vi "MA-K3BarcodeReader_Initialize.vi"(7 "Timeout(1000ms)":u32=1000, 8 "Error In":errorcluster, 11 "±½½X¾÷¦ê¤f":refnum<visa-resource-name>) -> (0 "Error Out":errorcluster, 3 "VISA Resource":refnum<visa-resource-name>)   [LabVIEW 2019]
uses:
  <vilib>/Instr/_visa.llb/VISA Configure Serial Port (Instr).vi
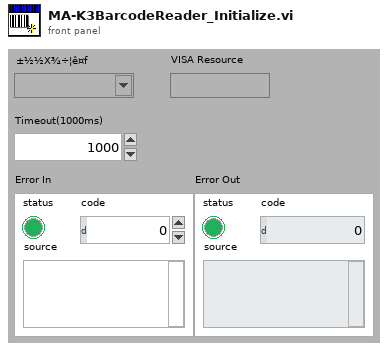
[diagram p1: front panel]
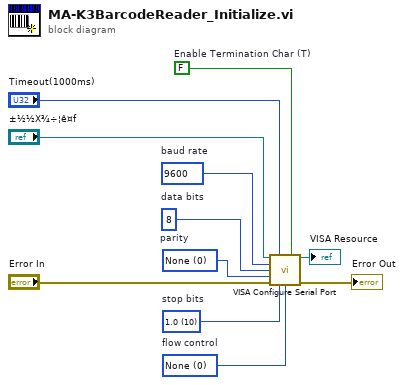
[diagram p0: block diagram]
diagram:
  w10 = u16 0 items=["None"=0, "XON/XOFF"=1, "RTS/CTS"=2, "DTR/DSR"=4]  # flow control
  w9 = u16 10 items=["1.0"=10, "1.5"=15, "2.0"=20]  # stop bits
  w7 = u16 0 items=["None", "Odd", "Even", "Mark", "Space"]  # parity
  w11 = u16 8  # data bits
  w6 = u32 9600  # baud rate
  w8 = FALSE  # Enable Termination Char (T)
  n1 = call-poly "VISA Configure Serial Port"("VISA resource name"="±½½X¾÷¦ê¤f", "timeout (10sec)"="Timeout(1000ms)", "Enable Termination\nChar (T)"=w8, "baud rate (9600)"=w6, "data bits (8)"=w11, "parity (0:none)"=w7, "error in (no error)"="Error In", "stop bits (10: 1 bit)"=w9, "flow control (0:none)"=w10) -> ("VISA resource name out"=→"VISA Resource":refnum<visa-resource-name>, "error out"=→"Error Out":errorcluster)  [unwired: 5 out]
